vi "AlarmOn FVG.vi"(7 "Mode":T1, 8 "Error In":errorcluster, 11 "Data In":bool) -> (0 "Error Out":errorcluster, 3 "Data Out":bool)   [LabVIEW 2014]
uses:
  Types/FVGFuncts.ctl
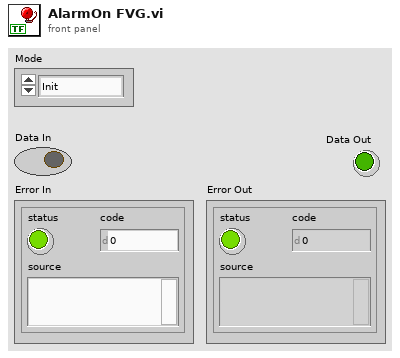
[diagram p1: front panel]
types:
  T1 = typedef "FVGFuncts.ctl" = enum16{"Init", "Set Data", "Get Data"}
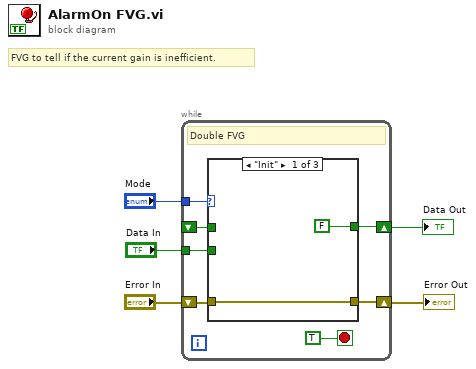
[diagram p0: block diagram]
diagram:
  # "FVG to tell if the current gain is inefficient."
  n1 = while {
    tunnel: "Mode" -> [w11]
    shift-right: [w6] -> w1
    shift-left: _ -> [w10]
    tunnel: "Data In" -> [w9]
    shift-right: [w7] -> w2
    shift-left: "Error In" -> [w8]
    stop <- TRUE stop-if-true
    # "Double FVG"
    n2 = case shown="\"Init\"" w11 {
      tunnel: w10 -> [_ _ w17]
      tunnel: w9 -> [_ w15 _]
      tunnel: w8 -> [w14 w16 w18]
      tunnel: [w14 w16 w18] -> w7
      tunnel: [FALSE w15 w17] -> w6
      frame "Init" {
      }
      frame "Set Data" {
      }
      frame "Get Data", Default {
      }
    }
  }
  "Data Out" <- w1
  "Error Out" <- w2
